vi "Execute.vi"(8 "error in (no error)":errorcluster, 11 "Command In":refnum<class "Command with Input.lvclass">) -> (0 "error out":errorcluster, 2 "Stop":bool, 3 "Command Out":refnum<class "Command with Input.lvclass">)   [LabVIEW 2017, in "Command Handler.lvlib" / "Command with Input.lvclass"]
uses:
  Command with Input.lvclass
  Command with Input.lvclass/Command with Input.ctl
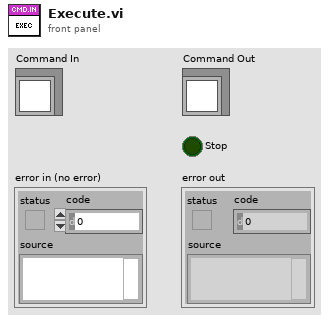
[diagram p1: front panel]
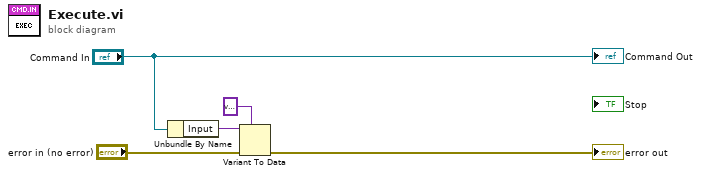
[diagram p0: block diagram]
diagram:
  n1 = Unbundle By Name("Command In") -> ("Input"=w2:variant)
  n2 = Variant To Data(error in="error in (no error)", type=variant, Variant=w2) -> (error out=→"error out":errorcluster)  [unwired: 1 out]
  "Command Out" <- "Command In"
